vi "5.3.vi"() -> ()   [LabVIEW 2023]
panel:
  in  "stop (T)":bool=TRUE
  out "Waveform Graph 2":dynamicdata(graph)
  out "Waveform Graph 1":dynamicdata(graph)
  in  "Forward":bool
  in  "Backward":bool
  in  "Duty Cycle (%)":dbl=50.0
  in  "stop":bool
  out "rps":dbl
  out "mps":dbl
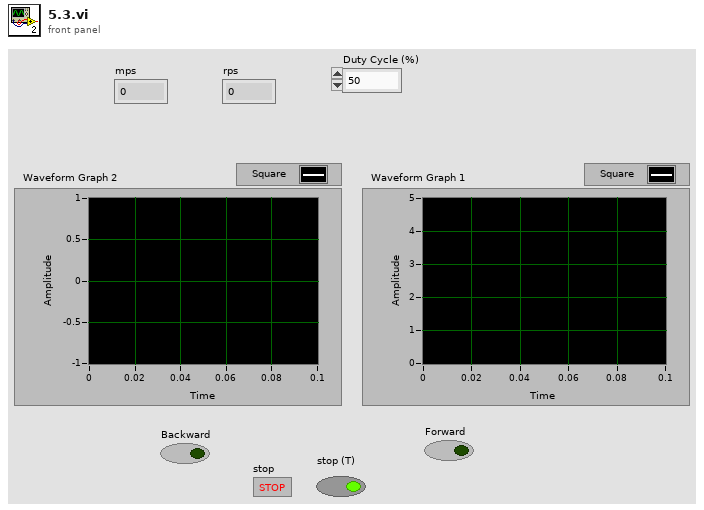
[diagram p1: front panel]
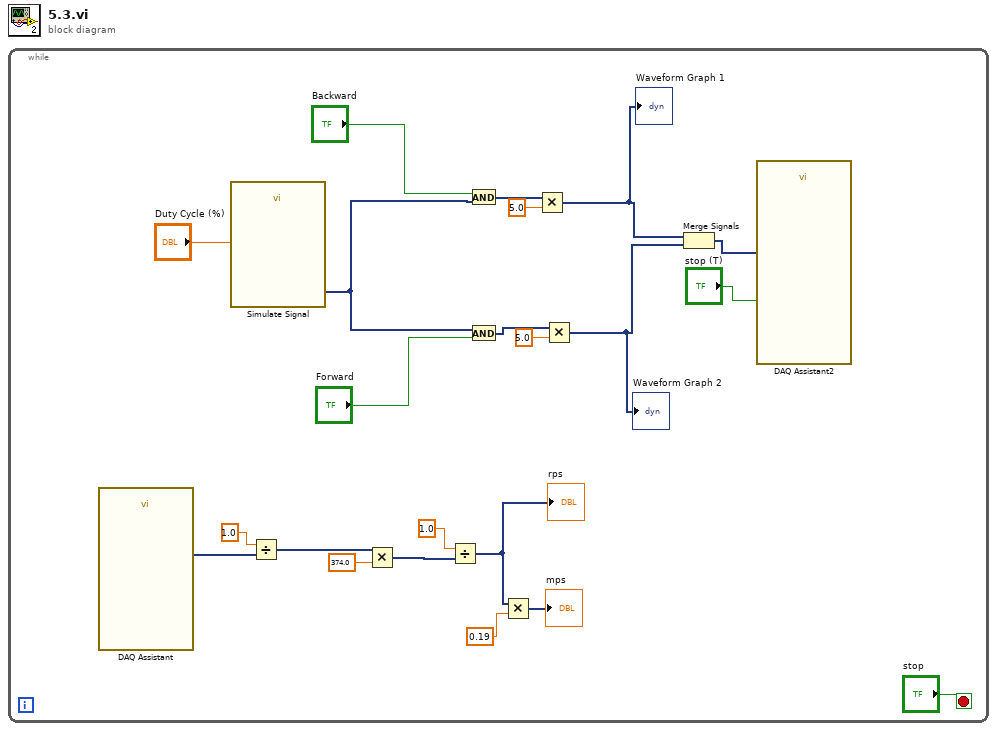
[diagram p0: block diagram]
diagram:
  n1 = while {
    stop <- "stop" stop-if-true
    n2 = call "DAQ Assistant"() -> ("data"=w22:dynamicdata)  [unwired: 17 in, 2 out]
    n3 = call "Simulate Signal"("Duty Cycle (%)"="Duty Cycle (%)") -> ("Square"=w10:dynamicdata)  [unwired: 13 in, 1 out]
    n4 = Divide(x=1.0, y=w22) -> (x/y=w20:dynamicdata)
    n5 = Multiply(x=w20, y=374.0) -> (x*y=w18:dynamicdata)
    n6 = Divide(x=1.0, y=w18) -> (x/y=w16:dynamicdata)
    "rps" <- w16
    n7 = And(x="Backward", y=w10) -> (x .and. y?=w8:dynamicdata)
    n8 = And(x=w10, y="Forward") -> (x .and. y?=w6:dynamicdata)
    n9 = Multiply(x=w16, y=0.19) -> (x*y=→"mps":dynamicdata)
    n10 = Multiply(x=w8, y=5.0) -> (x*y=w3:dynamicdata)
    "Waveform Graph 1" <- w3
    n11 = Multiply(x=w6, y=5.0) -> (x*y=w2:dynamicdata)
    "Waveform Graph 2" <- w2
    n12 = Merge Signals(w3, w2) -> (w1:dynamicdata)
    n13 = call "DAQ Assistant2"("data"=w1, "stop (T)"="stop (T)") -> ()  [unwired: 16 in, 2 out]
  }
